vi "Update Timer TIO.vi"(8 "error in (no error)":errorcluster, 10 "Timer Cluster":T1, 11 "task ID":u32 format="%.0x") -> (0 "error out":errorcluster, 2 "Timer Cluster Out":T1, 3 "Timer Value (s)":dbl format="%.2f")   [LabVIEW 2009]
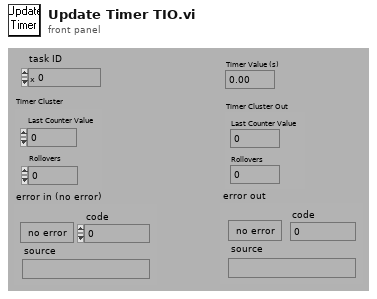
[diagram p1: front panel]
types:
  T1 = cluster{"Last Counter Value":u32, "Rollovers":i32}
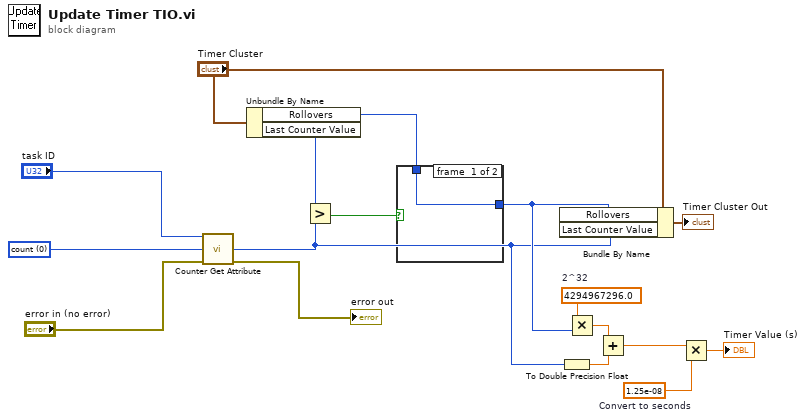
[diagram p0: block diagram]
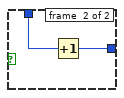
[diagram p2: hidden frame]
diagram:
  w12 = 4294967296.0  # 2^32
  w8 = 1.25e-08  # Convert to seconds
  w16 = u32 0 items=["count", "saved count", "count available", "available points", "armed", "TC reached", "done", "output state", "read mark", "write mark", "internal max timebase", "max prescale", "read mark high snapshot", "read mark low snapshot", "write mark high snapshot", "write mark low snapshot", "backlog high snapshot", "backlog low snapshot", "armed snapshot"] ("attribute ID")
  n1 = call <vilib>:"Counter Get Attribute.vi"("task ID"="task ID", "attribute ID"=w16, "error in (no error)"="error in (no error)") -> ("attribute value number"=w2:u32, "error out"=→"error out":errorcluster)  [unwired: 9 in, 2 out]
  n2 = Unbundle By Name("Timer Cluster") -> ("Rollovers"=w5:i32, "Last Counter Value"=w4:u32)
  n3 = Greater?(x=w4, y=w2) -> (0:w13:bool)
  n4 = case shown="True" w13 {
    tunnel: w5 -> [w18 w20]
    tunnel: [w18 w19] -> w3
    frame #0 {
    }
    frame #1 {
      n5 = Increment(x=w20) -> (x+1=w19:i32)
    }
  }
  n6 = Bundle By Name(cluster="Timer Cluster", "Rollovers"=w3, "Last Counter Value"=w2) -> (→"Timer Cluster Out":T1)
  n7 = To Double Precision Float(number=w2) -> (double precision float=w10:dbl)
  n8 = Multiply(x=w12, y=w3) -> (x*y=w11:dbl)
  n9 = Add(x=w11, y=w10) -> (x+y=w9:dbl)
  n10 = Multiply(x=w9, y=w8) -> (x*y=→"Timer Value (s)":dbl)
